vi "NXT_HINDBRAIN Write Data To Screen.vi"(2 "Clear Screen?":bool, 3 "_messageData":T2, 4 "_sensorData":T3, 5 "_motorCommands":T1={"_rudderCommand"=7, "_propCommand"=7, "_irServoCommand"=7}, 6 "NXT":T5) -> ()   [LabVIEW 2012, in "Tugboat.lvrbt"]
uses:
  Tugboat.lvrbt
  <vilib>/NXT/Subs/LVHSConnector.ctl
  sensorData_t.ctl
  irData_t.ctl
  messageData_t.ctl
  motorCommands_t.ctl
  <vilib>/NXT/Dual Mode Library/Display/drawText.vi
panel:
  # "L\nE\nF\nT"
  # "C\nE\nN\nT\nE\nR"
  # "R\nI\nG\nH\nT"
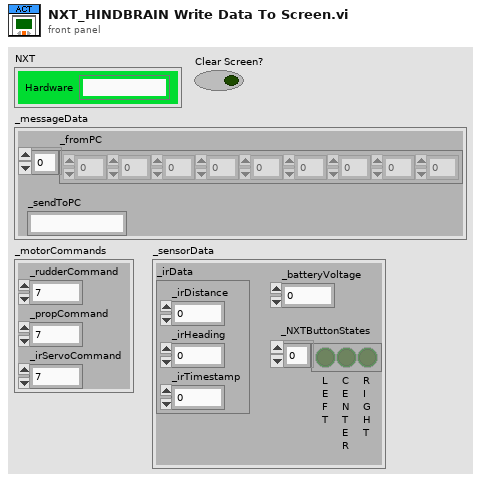
[diagram p1: front panel]
types:
  T1 = typedef "motorCommands_t.ctl" = cluster{"_rudderCommand":i8, "_propCommand":i8, "_irServoCommand":i8}
  T2 = typedef "messageData_t.ctl" = cluster{"_sendToPC":string, "_fromPC":u8[]}
  T3 = typedef "sensorData_t.ctl" = cluster{"_irData":T4, "_batteryVoltage":i32, "_NXTButtonStates":bool[]}
  T4 = typedef "irData_t.ctl" = cluster{"_irDistance":i32, "_irHeading":i32, "_irTimestamp":u32}
  T5 = typedef "LVHSConnector.ctl" = cluster{"Hardware":string, "Flattened String":string}
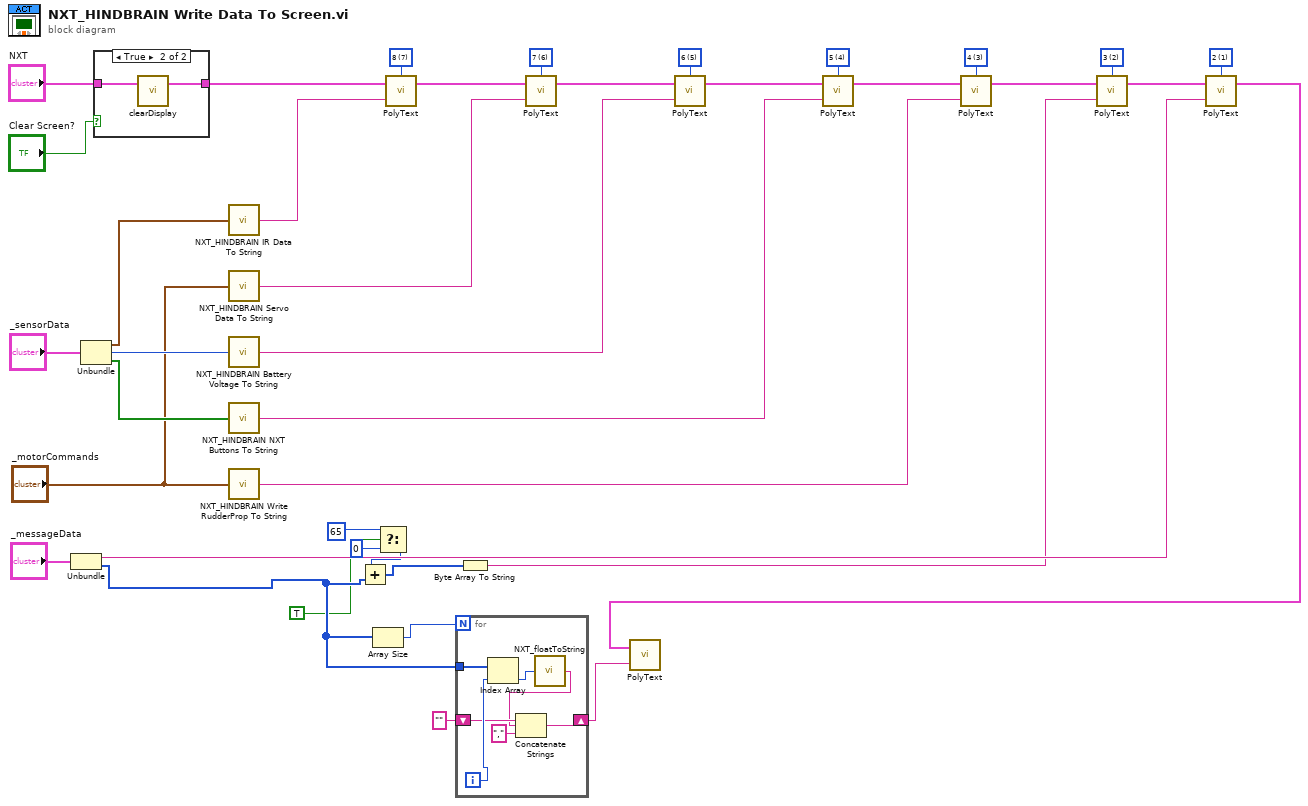
[diagram p0: block diagram]
diagram:
  w15 = i16 1 items=["1", "2", "3", "4", "5", "6", "7", "8"] ("Line")
  w17 = i16 2 items=["1", "2", "3", "4", "5", "6", "7", "8"] ("Line")
  w21 = i16 3 items=["1", "2", "3", "4", "5", "6", "7", "8"] ("Line")
  w25 = i16 4 items=["1", "2", "3", "4", "5", "6", "7", "8"] ("Line")
  w33 = i16 5 items=["1", "2", "3", "4", "5", "6", "7", "8"] ("Line")
  w35 = i16 6 items=["1", "2", "3", "4", "5", "6", "7", "8"] ("Line")
  w37 = i16 7 items=["1", "2", "3", "4", "5", "6", "7", "8"] ("Line")
  n1 = Unbundle("_messageData") -> ("_sendToPC"=w13:string, "_fromPC"=w6:u8[])
  n2 = Unbundle("_sensorData") -> ("_irData"=w31:T4, "_batteryVoltage"=w30:i32, "_NXTButtonStates"=w29:bool[])
  n3 = case shown="True" "Clear Screen?" {
    tunnel: "NXT" -> [w40 w42]
    tunnel: [w40 w41] -> w28
    frame False {
    }
    frame True {
      n4 = call <vilib>:"clearDisplay.vi"("NXT"=w42) -> ("NXT"=w41:T5)  [unwired: 3 in]
    }
  }
  n5 = call "NXT_HINDBRAIN IR Data To String.vi"("_irData"=w31) -> ("String"=w36:string)
  n6 = call "NXT_HINDBRAIN Servo Data To String.vi"("_motorCommands"="_motorCommands") -> ("String"=w34:string)
  n7 = call "NXT_HINDBRAIN Battery Voltage To String.vi"("_batteryVoltage"=w30) -> ("String"=w22:string)
  n8 = call "NXT_HINDBRAIN NXT Buttons To String.vi"("_NXTButtonStates"=w29) -> ("String"=w23:string)
  n9 = call "NXT_HINDBRAIN Write RudderProp To String.vi"("_motorCommands"="_motorCommands") -> ("String"=w19:string)
  n10 = Array Size(array=w6) -> (size(s)=w10:i32)
  n11 = Select(t=u8 65, s=TRUE, f=u8 0) -> (s? t:f=w2:u8)
  n12 = Add(x=w2, y=w6) -> (x+y=w1:u8[])
  n13 = call-poly <vilib>:"PolyText.vi"("Text"=w36, "NXT"=w28, "Line"=w37) -> ("NXT"=w27:T5)  [unwired: 1 in]
  n14 = for {
    N: w10 -> [_]
    tunnel: w6 -> [w49]
    shift-right: [w46] -> w8
    shift-left: "" -> [w47]
    i -> [w48]
    n15 = Index Array(array=w49, index=w48) -> (element=w45:u8)
    n16 = call <vilib>:"NXT_floatToString.vi"("number"=w45) -> ("string"=w44:string)
    n17 = Concatenate Strings(w47, w44, "," ("string")) -> (w46:string)
  }
  n18 = Byte Array To String(unsigned byte array=w1) -> (string=w11:string)
  n19 = call-poly <vilib>:"PolyText.vi"("Text"=w34, "NXT"=w27, "Line"=w35) -> ("NXT"=w26:T5)  [unwired: 1 in]
  n20 = call-poly <vilib>:"PolyText.vi"("Text"=w22, "NXT"=w26, "Line"=w33) -> ("NXT"=w24:T5)  [unwired: 1 in]
  n21 = call-poly <vilib>:"PolyText.vi"("Text"=w23, "NXT"=w24, "Line"=w25) -> ("NXT"=w20:T5)  [unwired: 1 in]
  n22 = call-poly <vilib>:"PolyText.vi"("Text"=w19, "NXT"=w20, "Line"=w21) -> ("NXT"=w16:T5)  [unwired: 1 in]
  n23 = call-poly <vilib>:"PolyText.vi"("Text"=w11, "NXT"=w16, "Line"=w17) -> ("NXT"=w14:T5)  [unwired: 1 in]
  n24 = call-poly <vilib>:"PolyText.vi"("Text"=w13, "NXT"=w14, "Line"=w15) -> ("NXT"=w9:T5)  [unwired: 1 in]
  n25 = call-poly <vilib>:"PolyText.vi"("Text"=w8, "NXT"=w9) -> ()  [unwired: 2 in, 1 out]
